vi "Read Message.vi"(8 "error in (no error)":errorcluster, 11 "RemoteControl in":refnum<class "RemoteControl.lvclass">) -> (0 "error out":errorcluster, 1 "Data":string, 2 "Command":string, 3 "RemoteControl out":refnum<class "RemoteControl.lvclass">, 4 "ID":string)   [LabVIEW 2019, in "RemoteControl.lvlib" / "RemoteControl.lvclass"]
uses:
  RemoteControl.lvclass
  RemoteControl.lvclass/RemoteControl.ctl
  Typedefs/Message--Cluster.ctl
  Private/RemoteControl.GlobalVariable.vi
  9449e617-4408-478f-b4f7-2d0bd89df068.vi
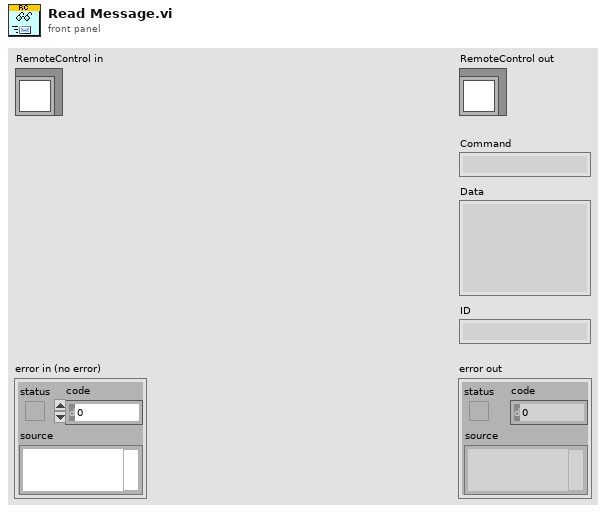
[diagram p1: front panel]
types:
  T1 = typedef "RemoteControl.lvlib/RemoteControl.lvclass/RC Process Type--Enum.ctl" = enum16{"Listener", "Server", "Client"}
  T2 = typedef "RemoteControl.lvlib/RemoteControl.lvclass/Message--Cluster.ctl" = cluster{"Command":string, "Data":variant, "ID":string}
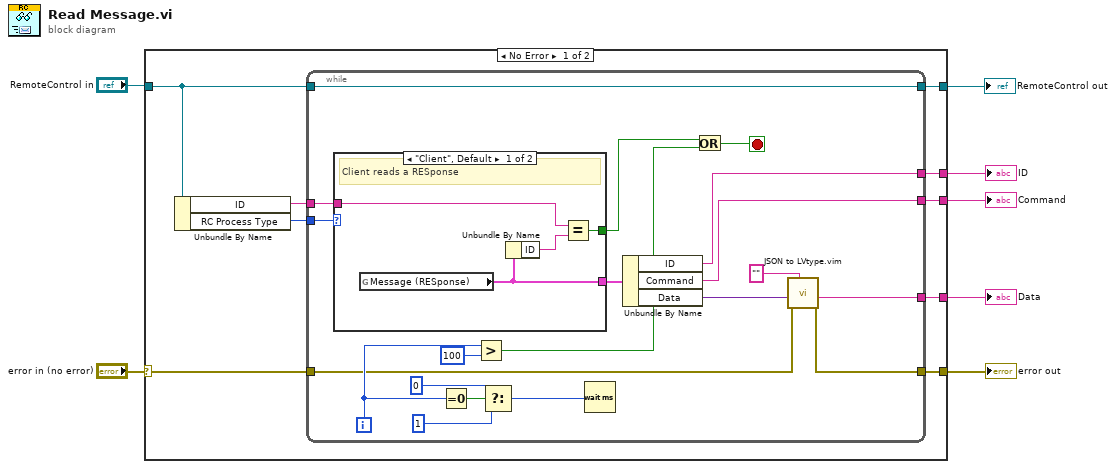
[diagram p0: block diagram]
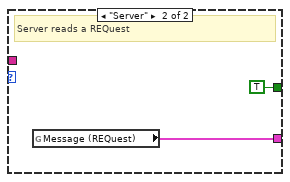
[diagram p2: hidden frame]
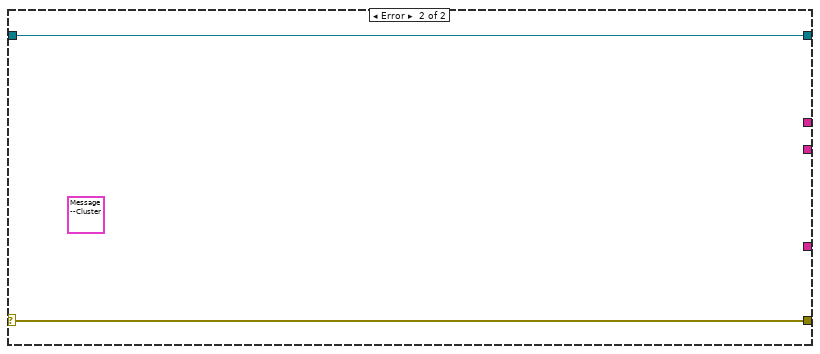
[diagram p3: hidden frame]
diagram:
  n1 = case shown="No Error" "error in (no error)" {
    selector: "error in (no error)" -> [w15 w43]
    tunnel: [w9 w44] -> w5
    tunnel: "RemoteControl in" -> [w8 w44]
    tunnel: [w16 _] -> w4
    tunnel: [w12 _] -> w3
    tunnel: [w11 _] -> w2
    tunnel: [w14 w43] -> w1
    frame No Error {
      n2 = Unbundle By Name(w8) -> ("ID"=w10:string, "RC Process Type"=w13:T1)
      n3 = while {
        tunnel: [w17] -> w16
        tunnel: w13 -> [w36]
        tunnel: [w33] -> w12
        tunnel: [w34] -> w11
        tunnel: w10 -> [w32]
        tunnel: w15 -> [w21]
        tunnel: [w20] -> w14
        tunnel: w8 -> [w19]
        tunnel: [w19] -> w9
        i -> [w27]
        stop <- w24 stop-if-true
        n4 = case shown="\"Client\", Default" w36 {
          tunnel: [w40 w42] -> w35
          tunnel: w32 -> [w37 _]
          tunnel: [w39 TRUE] -> w25
          frame "Client", Default {
            # "Client reads a RESponse"
            n5 = global read "RemoteControl.GlobalVariable.vi" "Message (RESponse)"() -> (w40:T2)
            n6 = Unbundle By Name(w40) -> ("ID"=w38:string)
            n7 = Equal?(x=w37, y=w38) -> (x = y?=w39:bool)
          }
          frame "Server" {
            # "Server reads a REQuest"
            n8 = global read "RemoteControl.GlobalVariable.vi" "Message (REQuest)"() -> (w42:T2)
          }
        }
        n9 = Equal To 0?(x=w27) -> (x = 0?=w31:bool)
        n10 = Greater?(x=w27, y=100) -> (0:w23:bool)
        n11 = Select(t=u32 0 ("milliseconds to wait"), s=w31, f=u32 1 ("milliseconds to wait")) -> (s? t:f=w28:u32)
        n12 = Wait (ms)(milliseconds to wait=w28) -> ()  [unwired: 1 out]
        n13 = Unbundle By Name(w35) -> ("ID"=w34:string, "Command"=w33:string, "Data"=w18:variant)
        n14 = Or(x=w25, y=w23) -> (x .or. y?=w24:bool)
        n15 = call "JSON to LVtype.vim"("type"="", "error in (no error)"=w21, "JSON Data in"=w18) -> ("error out"=w20:errorcluster, "Data out"=w17:string)  [unwired: 7 in]
      }
    }
    frame Error {
      (unwired) T2 {"Command"="", "Data"=variant(string ""), "ID"=""} ("Message")
    }
  }
  "error out" <- w1
  "RemoteControl out" <- w5
  "ID" <- w2
  "Command" <- w3
  "Data" <- w4
